vi "Erase Sequence (SubVI).vi"(0 "Refs":T1) -> ()   [LabVIEW 2010]
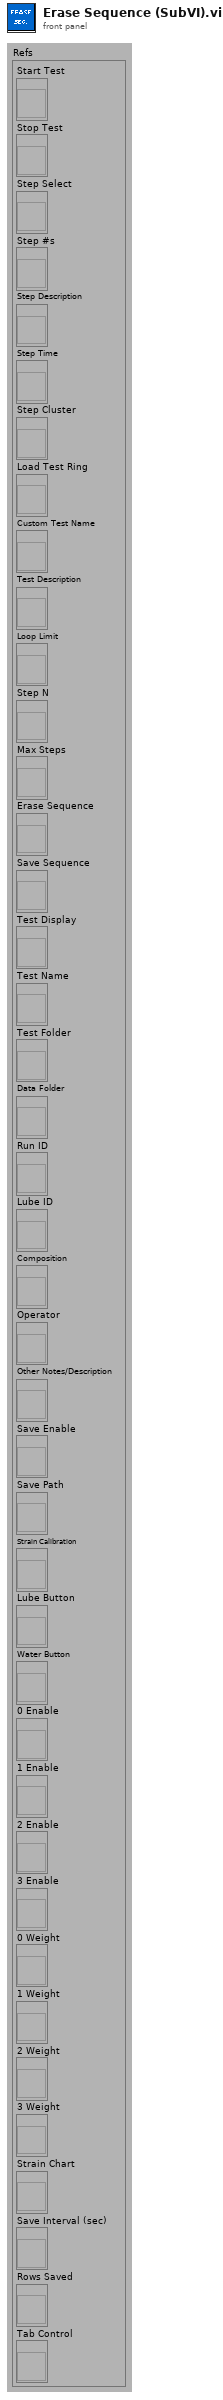
[diagram p1: front panel]
types:
  T1 = cluster{"Start Test":refnum<vi>, "Stop Test":refnum<vi>, "Step Select":refnum<vi>, "Step #s":refnum<vi>, "Step Description":refnum<vi>, "Step Time":refnum<vi>, "Step Cluster":refnum<vi>, "Load Test Ring":refnum<vi>, "Custom Test Name":refnum<vi>, "Test Description":refnum<vi>, "Loop Limit":refnum<vi>, "Step N":refnum<vi>, "Max Steps":refnum<vi>, "Erase Sequence":refnum<vi>, "Save Sequence":refnum<vi>, "Test Display":refnum<vi>, "Test Name":refnum<vi>, "Test Folder":refnum<vi>, "Data Folder":refnum<vi>, "Run ID":refnum<vi>, "Lube ID":refnum<vi>, "Composition":refnum<vi>, "Operator":refnum<vi>, "Other Notes/Description":refnum<vi>, "Save Enable":refnum<vi>, "Save Path":refnum<vi>, "Strain Calibration":refnum<vi>, "Lube Button":refnum<vi>, "Water Button":refnum<vi>, "0 Enable":refnum<vi>, "1 Enable":refnum<vi>, "2 Enable":refnum<vi>, "3 Enable":refnum<vi>, "0 Weight":refnum<vi>, "1 Weight":refnum<vi>, "2 Weight":refnum<vi>, "3 Weight":refnum<vi>, "Strain Chart":refnum<vi>, "Save Interval (sec)":refnum<vi>, "Rows Saved":refnum<vi>, "Tab Control":refnum<vi>}
  T2 = cluster{"Step Time Unit":u16, "Step End Action":u16, "Relay1":bool, "Relay2":bool}[]
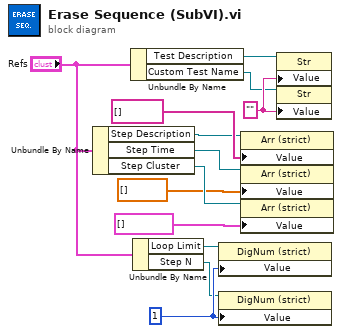
[diagram p0: block diagram]
diagram:
  w12 = ""
  w9 = 1
  n1 = Unbundle By Name("Refs") -> ("Step Description"=w1:refnum<vi>, "Step Time"=w3:refnum<vi>, "Step Cluster"=w5:refnum<vi>)
  n2 = Unbundle By Name("Refs") -> ("Test Description"=w10:refnum<vi>, "Custom Test Name"=w11:refnum<vi>)
  n3 = Unbundle By Name("Refs") -> ("Loop Limit"=w7:refnum<vi>, "Step N"=w8:refnum<vi>)
  n4 = property class="DigNum (strict)"(reference=w7, "Value"=w9) -> ()  [unwired: 1 in, 2 out]
  n5 = property class="DigNum (strict)"(reference=w8, "Value"=w9) -> ()  [unwired: 1 in, 2 out]
  n6 = property class="Arr (strict)"(reference=w1, "Value"=string[] []) -> ()  [unwired: 1 in, 2 out]
  n7 = property class="Arr (strict)"(reference=w3, "Value"=dbl[] []) -> ()  [unwired: 1 in, 2 out]
  n8 = property class="Arr (strict)"(reference=w5, "Value"=T2 []) -> ()  [unwired: 1 in, 2 out]
  n9 = property class="Str"(reference=w10, "Value"=w12) -> ()  [unwired: 1 in, 2 out]
  n10 = property class="Str"(reference=w11, "Value"=w12) -> ()  [unwired: 1 in, 2 out]
